vi "_EnqueueMessage.vi"(5 "In Front? (F)":bool, 7 "Timeout (-1 ms)":i32, 8 "error in (no error)":errorcluster, 10 "Message":refnum<class "Message.lvclass">, 11 "MessageQueue in":refnum<class "MessageQueue.lvclass">) -> (0 "error out":errorcluster, 3 "MessageQueue out":refnum<class "MessageQueue.lvclass">, 4 "Timed Out?":bool)   [LabVIEW 2013, in "LapDog.Messaging.v3.lvlib" / "MessageQueue.lvclass"]
doc: "This protected method is intended to be overridden by children of the MessageQueue class. This allows users to use the polymorphic EnqueueMessage method on the palette with the child object.\n\nAdds a message object to the queue. By default the message is added to the rear of the queue. Set 'In Front?' to TRUE to add the message to the front of the queue.\n\nThis method executes regardless of the error in state."
uses:
  MessageQueue.lvclass
  Message/Message.lvclass
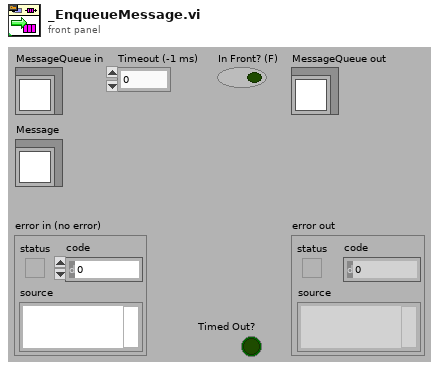
[diagram p1: front panel]
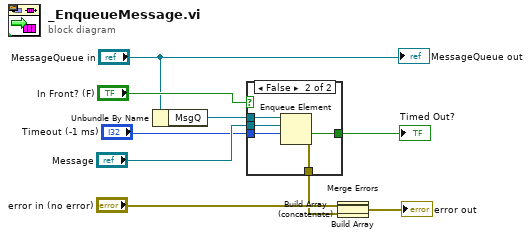
[diagram p0: block diagram]
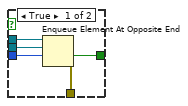
[diagram p2: hidden frame]
diagram:
  n1 = Unbundle By Name("MessageQueue in") -> ("MsgQ"=w5:refnum<queue>)
  n2 = case shown="False" "In Front? (F)" {
    tunnel: w5 -> [w16 w21]
    tunnel: [w15 w20] -> w7
    tunnel: "Message" -> [w14 w19]
    tunnel: "Timeout (-1 ms)" -> [w13 w18]
    tunnel: [w12 w17] -> w3
    frame True {
      n3 = Enqueue Element At Opposite End(queue=w16, element=w14, timeout in ms (-1)=w13) -> (timed out?=w12:bool, error out=w15:errorcluster)  [unwired: 1 in, 1 out]
    }
    frame False {
      n4 = Enqueue Element(queue=w21, element=w19, timeout in ms (-1)=w18) -> (timed out?=w17:bool, error out=w20:errorcluster)  [unwired: 1 in, 1 out]
    }
  }
  "Timed Out?" <- w3
  n5 = Build Array("error in (no error)", w7) -> (w2:errorcluster[])
  n6 = Build Array (concatenate)(w2) -> (w1:errorcluster[])
  n7 = Merge Errors(w1) -> (→"error out":errorcluster)
  "MessageQueue out" <- "MessageQueue in"
